vi "libAgLabviewPath.vi"(8 "Error In":errorcluster) -> (0 "Error Out":errorcluster, 3 "libAgLabview path":path)   [LabVIEW 2015]
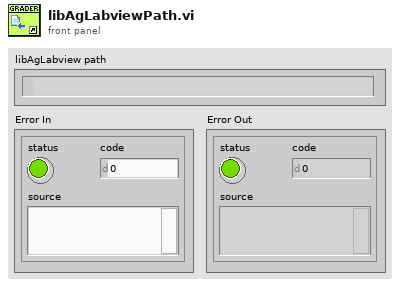
[diagram p1: front panel]
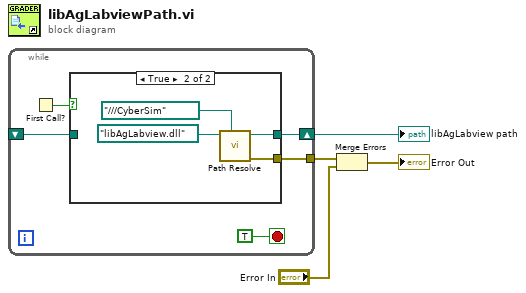
[diagram p0: block diagram]
diagram:
  n1 = while {
    shift-right: [w7] -> w4
    shift-left: _ -> [w5]
    tunnel: [w6] -> w3
    stop <- TRUE stop-if-true
    n2 = First Call?() -> (First Call?: T/F=w9:bool)
    n3 = case shown="True" w9 {
      tunnel: [_ w14] -> w6
      tunnel: [w10 w13] -> w7
      tunnel: w5 -> [w10 _]
      frame False {
      }
      frame True {
        n4 = call "Path Resolve.vi"("additional search path"=path "../../../CyberSim" ("base path"), "absolute or relative path"=path "libAgLabview.dll") -> ("Error Out"=w14:errorcluster, "resolved path"=w13:path)  [unwired: 8 in]
      }
    }
  }
  "libAgLabview path" <- w4
  n5 = Merge Errors(w3, "Error In") -> (→"Error Out":errorcluster)
